vi "_Remote Set PIC.vi"(4 "error in (no error)":errorcluster, 6 "Set Value":u32, 7 "PIC Channel":T1) -> (0 "error out":errorcluster, 2 "Received Value":u16, 3 "Received Header":u16)   [LabVIEW 2012]
uses:
  Type/_PIC Channel.ctl
  Type/_RT Command.ctl
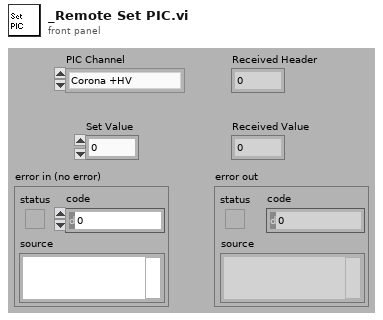
[diagram p1: front panel]
types:
  T1 = typedef "_PIC Channel.ctl" = enum16{"Corona +HV", "Corona -HV", "HSID Temp", "Time Const 1", "Curtain Cap +HV", "Curtain Cap -HV", "Time Const 2", "Source 1 +HV", "Source 1 -HV", "Source 1 Temp", "Time Const 3", "Source 2 +HV", "Source 2 -HV", "Source 2 Temp", "Time Const 4"}
  T2 = typedef "_RT Command.ctl" = enum16{"Start", "Stop", "Runtime Update", "Get Data", "Get Info", "Get Status", "Get Param", "Get Config", "Get Table", "Read ADC", "Set Oscillator", "Update Config", "Update Table", "Set All Pol", "Set Pol and DC", "Set Max Mass", "Toggle RP", "Toggle EL", "Set PIC", "Initialize Turbo", "Send Turbo Comm", "Close Turbo", "P1", "P2", "P3", "Send Serial", "Set LC Out", "Get LC In", "Read VAC", "Test Table", "Toggle Power", "Get Startup", "Set Startup", "Get ADC Table", "Set ADC Table", "Get Brief Status", "Get Detail Status", "Auxiliary Update", "Set CC Logics", "Set CC Input Logics", "Ignore Error"}
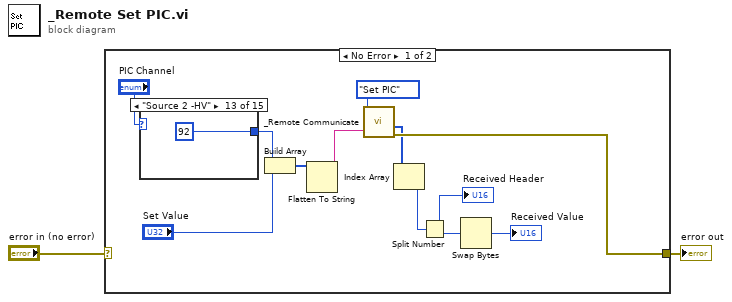
[diagram p0: block diagram]
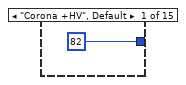
[diagram p2: hidden frame]
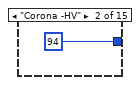
[diagram p3: hidden frame]
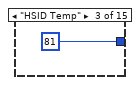
[diagram p4: hidden frame]
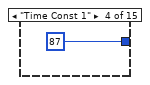
[diagram p5: hidden frame]
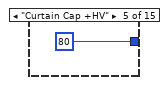
[diagram p6: hidden frame]
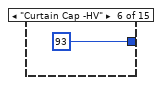
[diagram p7: hidden frame]
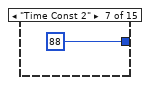
[diagram p8: hidden frame]
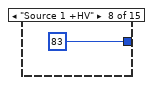
[diagram p9: hidden frame]
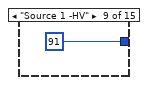
[diagram p10: hidden frame]
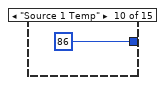
[diagram p11: hidden frame]
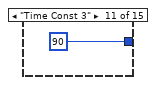
[diagram p12: hidden frame]
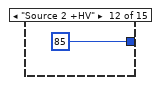
[diagram p13: hidden frame]
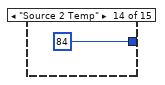
[diagram p14: hidden frame]
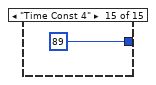
[diagram p15: hidden frame]
diagram:
  n1 = case shown="No Error" "error in (no error)" {
    selector: "error in (no error)" -> [_ w30]
    tunnel: [w7 w30] -> w1
    frame No Error {
      n2 = case shown="\"Source 2 -HV\"" "PIC Channel" {
        tunnel: [u32 82 u32 94 u32 81 u32 87 u32 80 u32 93 u32 88 u32 83 u32 91 u32 86 u32 90 u32 85 u32 92 u32 84 u32 89] -> w8
        frame "Corona +HV", Default {
        }
        frame "Corona -HV" {
        }
        frame "HSID Temp" {
        }
        frame "Time Const 1" {
        }
        frame "Curtain Cap +HV" {
        }
        frame "Curtain Cap -HV" {
        }
        frame "Time Const 2" {
        }
        frame "Source 1 +HV" {
        }
        frame "Source 1 -HV" {
        }
        frame "Source 1 Temp" {
        }
        frame "Time Const 3" {
        }
        frame "Source 2 +HV" {
        }
        frame "Source 2 -HV" {
        }
        frame "Source 2 Temp" {
        }
        frame "Time Const 4" {
        }
      }
      n3 = Build Array(w8, "Set Value") -> (w10:u32[])
      n4 = Flatten To String(anything=w10) -> (data string=w11:string)  [unwired: 1 in, 4 out]
      n5 = call "_Remote Communicate.vi"("String"=w11, "Command"=_RT_Command."Set PIC") -> ("error out"=w7:errorcluster, "Data Array"=w3:i32[])  [unwired: 4 in, 2 out]
      n6 = Index Array(array=w3) -> (element=w5:i32)  [unwired: 1 in]
      n7 = Split Number(x=w5) -> (hi(x)=→"Received Header":u16, lo(x)=w12:u16)
      n8 = Swap Bytes(anything=w12) -> (byte swapped=→"Received Value":u16)
    }
    frame Error {
    }
  }
  "error out" <- w1
